vi "DAQ.44xx.MIN MAX Fs.vi"(8 "error in (no error)":errorcluster, 11 "task []":refnum<k21>[](array[refnum])) -> (0 "error out":errorcluster, 1 "Max(SampClk.MinRate) (S/s)":dbl, 2 "Min(SampClk.MaxRate) (S/s)":dbl)   [LabVIEW 2019, in "Instrument.Lockin.lvlib" / "Instrument.DAQ.lvclass"]
doc: "Calculates the smallest maximum sample rate among all synchronized devices"
uses:
  Instrument.DAQ.lvclass
  <resource>/objmgr/daqmx.rc
panel:
  out "Fs (S/s)":dbl[](array[numeric]) format="%#_13g"
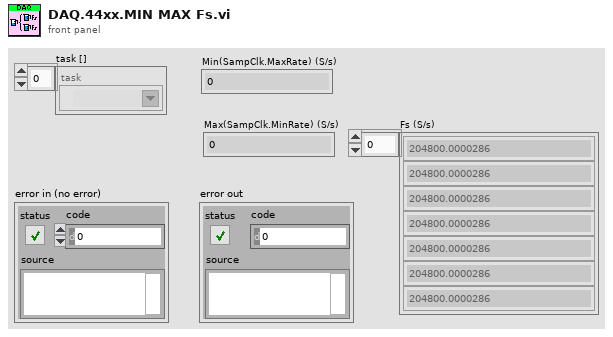
[diagram p1: front panel]
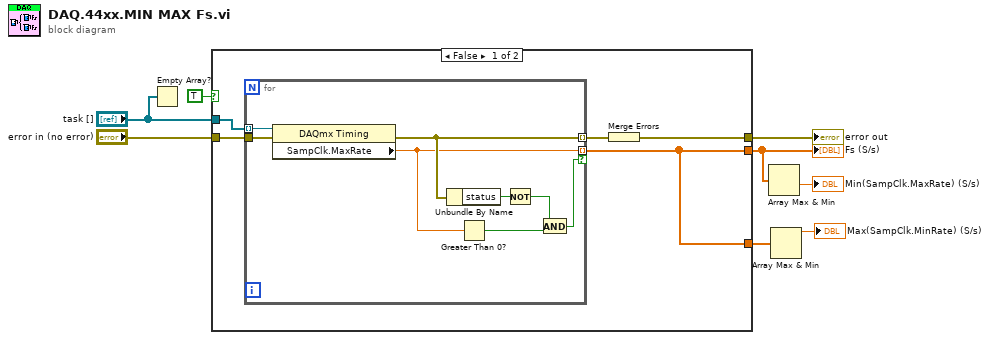
[diagram p0: block diagram]
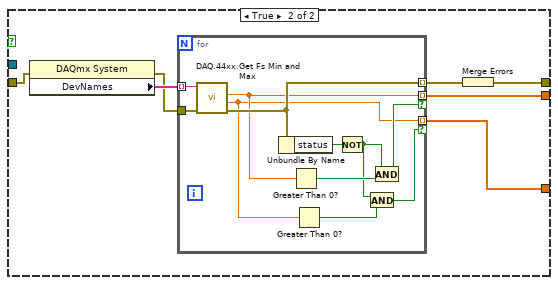
[diagram p2: hidden frame]
diagram:
  n1 = Empty Array?(array="task []") -> ()  [unwired: 1 out]
  n2 = case shown="False" TRUE {
    tunnel: [w10 w25] -> w8
    tunnel: "error in (no error)" -> [w13 w27]
    tunnel: [w9 w26] -> w5
    tunnel: "task []" -> [w12 _]
    tunnel: [w9 w22] -> w3
    frame False {
      n3 = for {
        tunnel: [w17] -> w9 mode=indexing if=w14
        tunnel: w13 -> [w21]
        tunnel: w12 -> [w20] mode=indexing
        tunnel: [w18] -> w11 mode=indexing
        n4 = property class="DAQmx Timing"(reference=w20, error in=w21) -> (error out=w18:errorcluster, "SampClk.MaxRate"=w17:dbl)  [unwired: 1 out]
        n5 = Unbundle By Name(w18) -> ("status"=w19:bool)
        n6 = Greater Than 0?(x=w17) -> (x > 0?=w16:bool)
        n7 = Not(x=w19) -> (.not. x?=w15:bool)
        n8 = And(x=w15, y=w16) -> (x .and. y?=w14:bool)
      }
      n9 = Merge Errors(w11) -> (w10:errorcluster)
    }
    frame True {
      n10 = property class="DAQmx System"(error in=w27) -> (error out=w24:errorcluster, "DevNames"=w28:tag[])  [unwired: 1 in, 1 out]
      n11 = for {
        tunnel: w28 -> [w39] mode=indexing
        tunnel: w24 -> [w38]
        tunnel: [w33] -> w26 mode=indexing if=w35
        tunnel: [w34] -> w23 mode=indexing
        tunnel: [w30] -> w22 mode=indexing if=w29
        n12 = call "DAQ.44xx.Get Fs Min and Max.vi"("error in (no error)"=w38, "DAQmx Device Name"=w39) -> ("error out"=w34:errorcluster, "Fs Min"=w30:dbl, "Fs Max"=w33:dbl)  [unwired: 7 in]
        n13 = Unbundle By Name(w34) -> ("status"=w37:bool)
        n14 = Greater Than 0?(x=w33) -> (x > 0?=w36:bool)
        n15 = Greater Than 0?(x=w30) -> (x > 0?=w32:bool)
        n16 = Not(x=w37) -> (.not. x?=w31:bool)
        n17 = And(x=w31, y=w32) -> (x .and. y?=w29:bool)
        n18 = And(x=w31, y=w36) -> (x .and. y?=w35:bool)
      }
      n19 = Merge Errors(w23) -> (w25:errorcluster)
    }
  }
  "error out" <- w8
  "Fs (S/s)" <- w5
  n20 = Array Max & Min(array=w5) -> (min value=→"Min(SampClk.MaxRate) (S/s)":dbl)  [unwired: 3 out]
  n21 = Array Max & Min(array=w3) -> (max value=→"Max(SampClk.MinRate) (S/s)":dbl)  [unwired: 3 out]
